vi "Base64 to Picture.vi"(8 "error in (no error)":errorcluster, 10 "Base64 PNG Data":string) -> (0 "error out":errorcluster, 2 "Picture":picture)   [LabVIEW 2020, in "VolatusGUIEditorCore.lvlib"]
uses:
  VolatusGUIEditorCore.lvlib
  lv-web-crypto/lv-base64/Base64.lvlib
  <vilib>/picture/picture.llb/imagedata.ctl
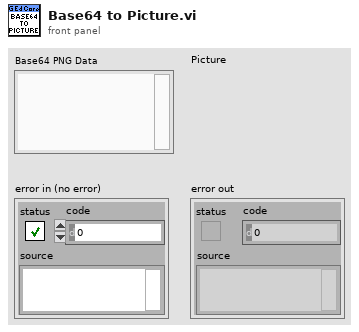
[diagram p1: front panel]
types:
  T1 = typedef "imagedata.ctl" = cluster{"image type":i32, "image depth":i32, "image":u8[], "mask":u8[], "colors":u32[], "Rectangle":cluster{"left":i16, "top":i16, "right":i16, "bottom":i16}}
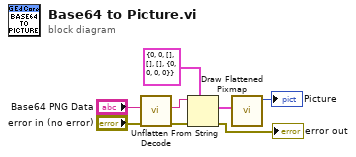
[diagram p0: block diagram]
diagram:
  n1 = call "Decode.vi"("error in (no error)"="error in (no error)", "string in (base64-encoded)"="Base64 PNG Data") -> ("error out"=w3:errorcluster, "string out (decoded)"=w4:string)  [unwired: 8 in]
  n2 = Unflatten From String(type=T1 {"image type"=0, "image depth"=0, "image"=[], "mask"=[], "colors"=[], "Rectangle"={"left"=0, "top"=0, "right"=0, "bottom"=0}} ("image data"), binary string=w4, error in (no error)=w3) -> (value=w2:T1, error out=→"error out":errorcluster)  [unwired: 2 in, 1 out]
  n3 = call <vilib>:"Draw Flattened Pixmap.vi"("image data"=w2) -> ("new picture"=→"Picture":picture)  [unwired: 8 in]
